vi "G# - InterfaceDemo.vi"() -> ()   [LabVIEW 2017]
doc: "G# Interface Implementation\nThis examples demonstrates how to use the G#Interface. The interface concept is an alternative design principle to multiple inheritance (just as in C# and Java). Classes that are not related can implement the same interface and the reference of the interface could be treated just as they are from the same class.\n\nBy using the G# Debugger found in Tools->G# Debugger a text log can be followed showing how the objects were created and destroyed."
uses:
  IMyInterface_interface/IMyInterface.lvclass
  C:/Program Files (x86)/National Instruments/LabVIEW 2017/vi.lib/addons/_AddQ/G#Object/G#Object.lvclass
  MyClass1_class/MyClass1.lvclass
  MyClass2_class/MyClass2.lvclass
  MyClass2_class/MyClass2_IMyInterface/MyClass2_IMyInterface.lvclass
  C:/Project/G#Utveckling/trunk/G# Framework/examples/AddQ/G#/Interface/IMyInterface_interface/IMyInterface.lvclass
  MyClass1_class/MyClass1_IMyInterface/MyClass1_IMyInterface.lvclass
  vi.lib/addons/_AddQ/G#Object/G#Object.lvclass
panel:
  out "# of objects killed":i32
  out "OK":bool
  in  "error in (no error)":errorcluster
  out "MyClass2 is instance of IMyInterface":bool
  out "MyClass1 is instance of IMyInterface":bool
  out "error out":errorcluster
  out "Class Name":string[](array[string])
  # "G# Interface Implementation with wrapper classes.\nThis examples demonstrates how to use the G#Interface with wrapper classes. The interface concept is an alternative design principle to multiple inheritance (just as in C# and Java).\nClasses that are not related can implement the same interface and the reference of the interface could be treated just as they are from the same class.\n\nBy using the G# Debugger found in Tools->G# Debugger a text log can be followed showing how the objects were created and destroyed."
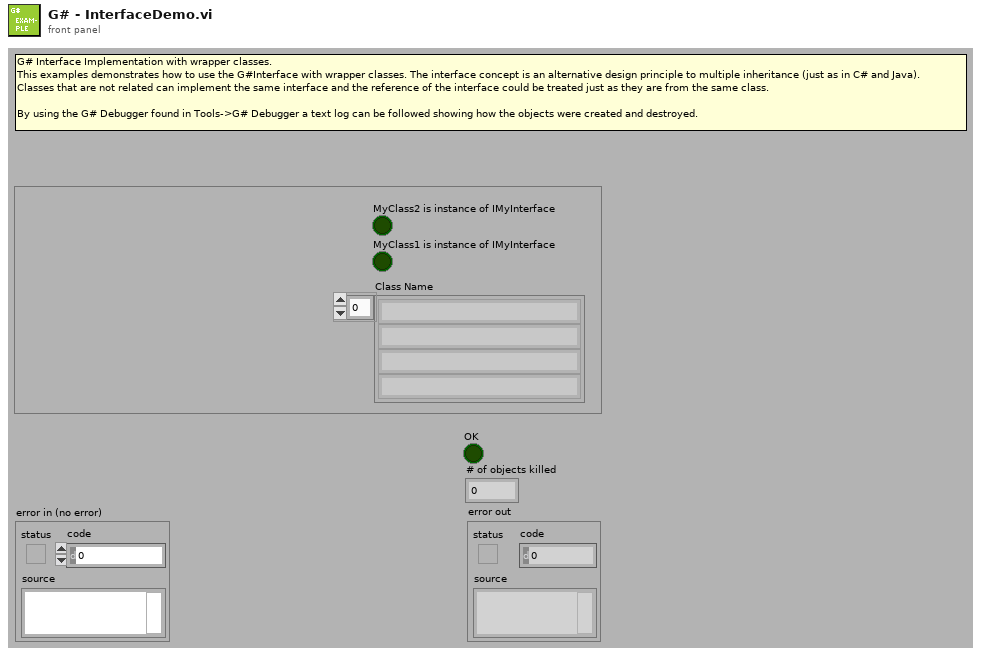
[diagram p1: front panel]
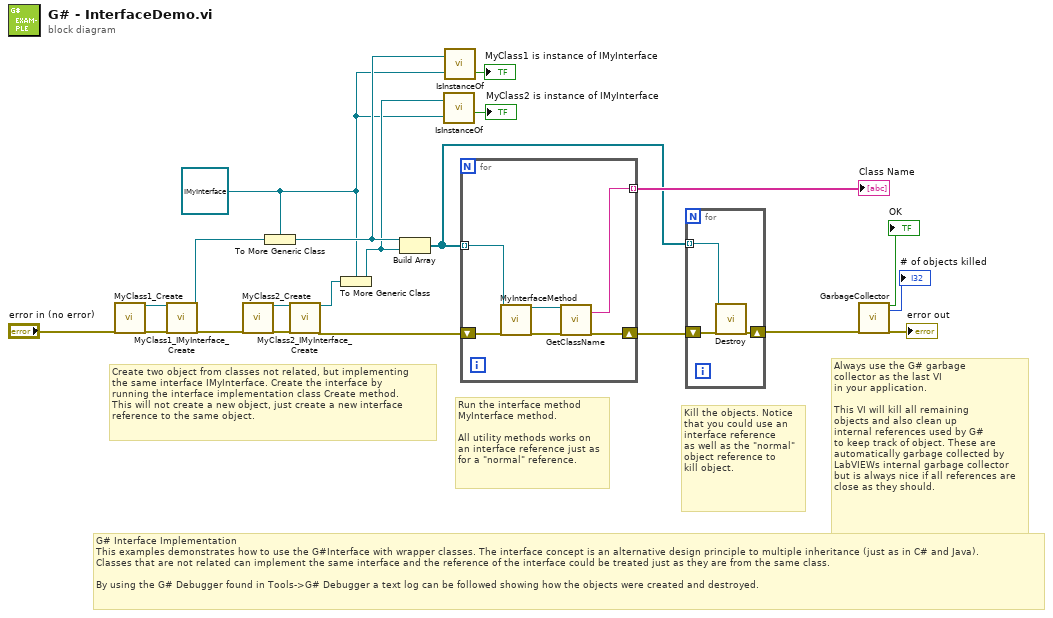
[diagram p0: block diagram]
diagram:
  w4 = refnum<class "IMyInterface.lvclass"> refnum ("IMyInterface.lvclass")
  # "G# Interface Implementation\nThis examples demonstrates how to use the G#Interface with wrapper classes. The interface concept is an alternative design principle to multiple inheritance (just as in C# and Java).\nClasses that are not related can implement the same interface and the reference of the interface could be treated just as they are from the same class.\n\nBy using the G# Debugger found in Tools->G# Debugger a text log can be followed showing how the objects were created and destroyed."
  # "Always use the G# garbage\ncollector as the last VI\nin your application.\n\nThis VI will kill all remaining\nobjects and also clean up\ninternal references used by G#\nto keep track of object. These are\nautomatically garbage collected by\nLabVIEWs internal garbage collector\nbut is always nice if all references are\nclose as they should."
  # "Kill the objects. Notice\nthat you could use an\ninterface reference\nas well as the \"normal\"\nobject reference to\nkill object."
  # "Run the interface method\nMyInterface method.\n\nAll utility methods works on\nan interface reference just as\nfor a \"normal\" reference."
  # "Create two object from classes not related, but implementing\nthe same interface IMyInterface. Create the interface by\nrunning the interface implementation class Create method.\nThis will not create a new object, just create a new interface\nreference to the same object."
  n1 = call "MyClass1_Create.vi"("error in (no error)"="error in (no error)") -> ("reference out"=w8:refnum<class "MyClass1.lvclass">, "error out"=w21:errorcluster)  [unwired: 17 in]
  n2 = call "MyClass1_IMyInterface_Create.vi"("reference in"=w8, "error in (no error)"=w21) -> ("reference out"=w18:refnum<class "MyClass1_IMyInterface.lvclass">, "error out"=w20:errorcluster)  [unwired: 16 in]
  n3 = call "MyClass2_Create.vi"("error in (no error)"=w20) -> ("reference out"=w9:refnum<class "MyClass2.lvclass">, "error out"=w19:errorcluster)  [unwired: 17 in]
  n4 = To More Generic Class(target class=w4, reference=w18) -> (generic class reference=w7:refnum<class "IMyInterface.lvclass">)
  n5 = call "MyClass2_IMyInterface_Create.vi"("reference in"=w9, "error in (no error)"=w19) -> ("reference out"=w17:refnum<class "MyClass2_IMyInterface.lvclass">, "error out"=w16:errorcluster)  [unwired: 16 in]
  n6 = To More Generic Class(target class=w4, reference=w17) -> (generic class reference=w5:refnum<class "IMyInterface.lvclass">)
  n7 = Build Array(w7, w5) -> (w11:refnum<class "IMyInterface.lvclass">[])
  n8 = call-dynamic "IsInstanceOf.vi"("is object instance of"=w4, "reference in"=w5) -> ("is instance of"=→"MyClass2 is instance of IMyInterface":bool)  [unwired: 1 out]
  n9 = call-dynamic "IsInstanceOf.vi"("is object instance of"=w4, "reference in"=w7) -> ("is instance of"=→"MyClass1 is instance of IMyInterface":bool)  [unwired: 1 out]
  n10 = for {
    shift-right: [w24] -> w14
    shift-left: w16 -> [w27]
    tunnel: w11 -> [w26] mode=indexing
    tunnel: [w22] -> w13 mode=indexing
    n11 = call-dynamic "MyInterfaceMethod.vi"("reference in"=w26, "error in (no error)"=w27) -> ("reference out"=w23:refnum<class "IMyInterface.lvclass">, "error out"=w25:errorcluster)  [unwired: 16 in]
    n12 = call-dynamic "GetClassName.vi"("reference in"=w23, "error in (no error)"=w25) -> ("class name"=w22:string, "error out"=w24:errorcluster)  [unwired: 13 in, 3 out]
  }
  "Class Name" <- w13
  n13 = for {
    shift-right: [w29] -> w12
    shift-left: w14 -> [w30]
    tunnel: w11 -> [w28] mode=indexing
    n14 = call-dynamic "Destroy.vi"("reference in"=w28, "error in (no error)"=w30) -> ("error out"=w29:errorcluster)  [unwired: 16 in, 1 out]
  }
  n15 = call "GarbageCollector.vi"("error in (no error)"=w12) -> ("OK"=→"OK":bool, "# of objects killed"=→"# of objects killed":i32, "error out"=→"error out":errorcluster)  [unwired: 16 in]
